vi "Vision Processing.vi"(4 "error in (no error)":errorcluster, 7 "Image Size":T5=enum."320x240") -> ()   [LabVIEW 2016]
doc: "This VI runs in parallel to other tasks. It gets images from the camera, processes them for color or shape and use that information to affect robot behavior."
uses:
  <vilib>/Rock Robotics/WPI/Camera/WPI_CameraImageSize.ctl
  Quick Vision/Typedefs/typedef_enum_ColorSpace.ctl
  <vilib>/Rock Robotics/WPI/Camera/WPI_CameraWhite Balance Values.ctl
  <vilib>/Rock Robotics/WPI/Camera/WPI_CameraExposure Values.ctl
  <vilib>/Rock Robotics/WPI/Camera/WPI_CameraFrameRate.ctl
  Robot Global Data.vi
panel:
  in  "Frame Rate (fps)":T1=15
  in  "Brightness":i32=50
  in  "Compression":i32=40
  in  "Exposure":T2=enum."Flicker-free 60 Hz"
  in  "White Balance":T3=enum."Fixed fluorescent 1"
  in  "ColorMask Low/High":u8[][](array[slide])=[[0, 124], [155, 255], [178, 245]] scale=0.0..255.0
  in  "Threshhold":i32=20
  in  "ColorSpace":T4
  out "Process FPS":dbl=7.231066612610667 format="%.1f"
  # "Modify Values\n\nthen\n\nEdit (menu):\n\nMake Current\nValues Default"
  # "Red\nHue\n\n\n\nGrn\nSat\n\n\n\nBlu\nLit"
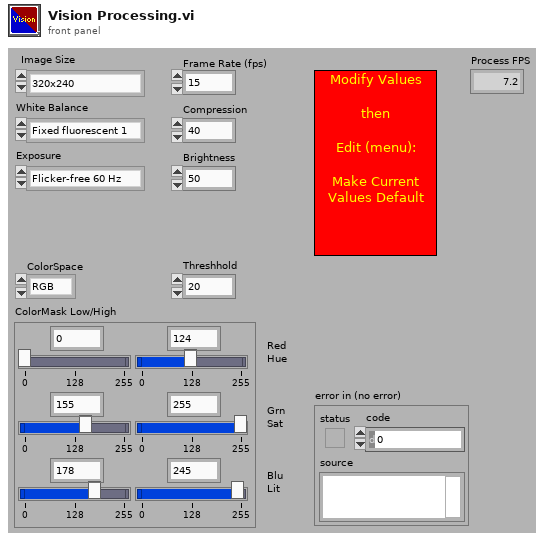
[diagram p1: front panel]
types:
  T1 = typedef "WPI_CameraFrameRate.ctl" = u32
  T2 = typedef "WPI_CameraExposure Values.ctl" = enum16{"Auto", "Flicker-free 50 Hz", "Flicker-free 60 Hz", "Hold current", "Custom"}
  T3 = typedef "WPI_CameraWhite Balance Values.ctl" = enum16{"Auto", "Fixed indoor", "Fixed outdoor 1", "Fixed outdoor 2", "Fixed fluorescent 1", "Fixed fluorescent 2", "Hold current", "Custom"}
  T4 = typedef "typedef_enum_ColorSpace.ctl" = enum16{"RGB", "HSL"}
  T5 = typedef "WPI_CameraImageSize.ctl" = enum16{"640x480", "320x240", "160x120", "Custom"}
  T6 = typedef "Image Type" = u32
  T7 = typedef "WPI_CameraDevRef.ctl" = cluster{"Camera Address":string, "CameraStatus":errorcluster}
  T8 = typedef "IMAQ Image.ctl" = refnum<image>
  T9 = typedef "typedef_cluster_Object Params.ctl" = cluster{"Dist_ft":dbl, "Deg_Rt":dbl, "Deg_Up":dbl, "Cam_FPS":dbl}
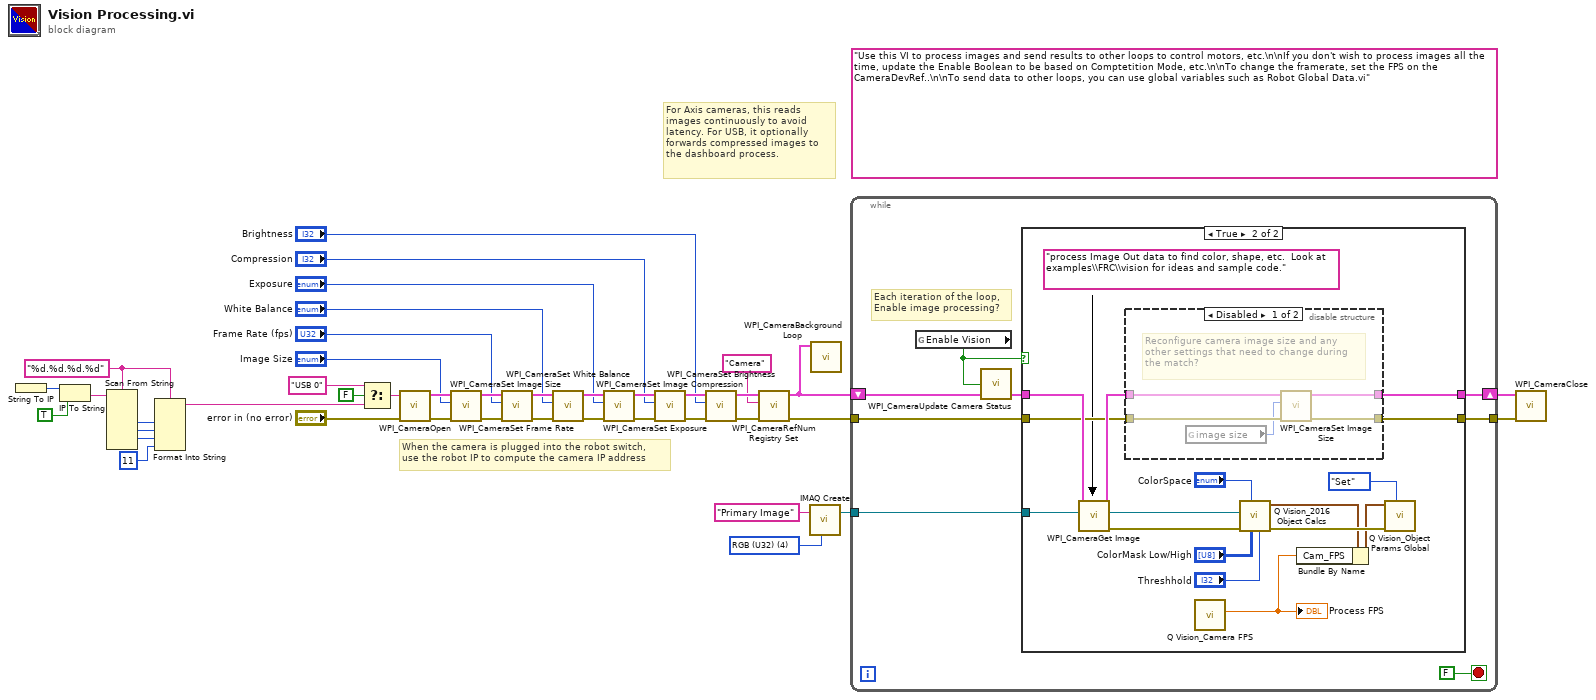
[diagram p0: block diagram]
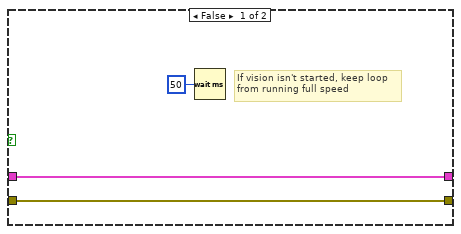
[diagram p2: hidden frame]
diagram:
  w14 = "%d.%d.%d.%d" ("format string")
  (unwired) "Use this VI to process images and send results to other loops to control motors, etc.\n\nIf you don't wish to process images all the time, update the Enable Boolean to be based on Comptetition Mode, etc.\n\nTo change the framerate, set the FPS on the CameraDevRef..\n\nTo send data to other loops, you can use global variables such as Robot Global Data.vi"
  w41 = T6 4 items=["Grayscale (U8)", "Grayscale (I16)", "Grayscale (SGL)", "Complex (CSG)", "RGB (U32)", "HSL (U32)", "RGB (U64)"] ("Image Type")
  # "When the camera is plugged into the robot switch,\nuse the robot IP to compute the camera IP address"
  # "For Axis cameras, this reads\nimages continuously to avoid\nlatency. For USB, it optionally\nforwards compressed images to\nthe dashboard process."
  n1 = String To IP() -> (0:w21:u32)  [unwired: 1 in]
  n2 = IP To String(1:TRUE ("dot notation? (F)"), 2:w21) -> (0:w19:string)
  n3 = Scan From String(format string=w14, input string=w19) -> (output 1=w18:i32, output 2=w17:i32, output 3=w16:i32)  [unwired: 7 in, 3 out]
  n4 = Format Into String(format string=w14, w18, w17, w16, 11 ("Compression")) -> (resulting string=w9:string)  [unwired: 2 in, 1 out]
  n5 = Select(t="USB 0" ("format string"), s=FALSE ("dot notation? (F)"), f=w9) -> (s? t:f=w7:string)
  n6 = call <vilib>:"WPI_CameraOpen.vi"("error in (no error)"="error in (no error)", "Camera Address"=w7) -> ("error out"=w32:errorcluster, "CameraDevRef"=w33:T7)  [unwired: 8 out]
  n7 = call <vilib>:"WPI_CameraSet Image Size.vi"("error in (no error)"=w32, "Image Size"="Image Size", "CameraDevRef"=w33) -> ("error out"=w31:errorcluster, "CameraDevRef Out"=w34:T7)  [unwired: 1 in, 6 out]
  n8 = call <vilib>:"WPI_CameraSet Frame Rate.vi"("error in (no error)"=w31, "Frame Rate (fps)"="Frame Rate (fps)", "CameraDevRef"=w34) -> ("error out"=w30:errorcluster, "CameraDevRef Out"=w36:T7)  [unwired: 7 out]
  n9 = call <vilib>:"WPI_CameraSet White Balance.vi"("error in (no error)"=w30, "White Balance"="White Balance", "CameraDevRef"=w36) -> ("error out"=w29:errorcluster, "CameraDevRef Out"=w35:T7)  [unwired: 1 in, 6 out]
  n10 = call <vilib>:"WPI_CameraSet Exposure.vi"("error in (no error)"=w29, "Exposure"="Exposure", "CameraDevRef"=w35) -> ("error out"=w28:errorcluster, "CameraDevRef Out"=w38:T7)  [unwired: 1 in, 6 out]
  n11 = call <vilib>:"WPI_CameraSet Image Compression.vi"("error in (no error)"=w28, "Compression"="Compression", "CameraDevRef"=w38) -> ("error out"=w27:errorcluster, "CameraDevRef Out"=w37:T7)  [unwired: 7 out]
  n12 = call <vilib>:"WPI_CameraSet Brightness.vi"("error in (no error)"=w27, "Brightness"="Brightness", "CameraDevRef"=w37) -> ("error out"=w25:errorcluster, "CameraDevRef Out"=w26:T7)  [unwired: 7 out]
  n13 = call <vilib>:"WPI_CameraRefNum Registry Set.vi"("error in (no error)"=w25, "refnum name"="Camera", "CameraDevRef"=w26) -> ("error out"=w6:errorcluster, "CameraDevRef"=w13:T7)  [unwired: 1 in, 6 out]
  n14 = call "IMAQ Create"("Image Name"="Primary Image", "Image Type"=w41) -> ("New Image"=w39:T8)  [unwired: 2 in, 2 out]
  n15 = call <vilib>:"WPI_CameraBackground Loop.vi"("CameraDevRef"=w13) -> ()  [unwired: 11 in]
  n16 = while {
    shift-right: [w49] -> w11
    shift-left: w13 -> [w47]
    tunnel: w39 -> [w48]
    tunnel: w6 -> [w44]
    tunnel: [w43] -> w5
    stop <- FALSE stop-if-true
    # "Each iteration of the loop,\nEnable image processing?"
    n17 = global read "Robot Global Data.vi" "Enable Vision"() -> (w45:bool)
    n18 = call <vilib>:"WPI_CameraUpdate Camera Status.vi"("CameraDevRef In"=w47, "Enable Vision"=w45) -> ("CameraDevRef Out"=w46:T7)  [unwired: 3 in]
    n19 = case shown="True" w45 {
      tunnel: w48 -> [_ w67]
      tunnel: [w52 w68] -> w49
      tunnel: w46 -> [w52 w66]
      tunnel: w44 -> [w50 w53]
      tunnel: [w50 w54] -> w43
      frame False {
        # "If vision isn't started, keep loop\nfrom running full speed"
        n20 = Wait (ms)(milliseconds to wait=u32 50) -> ()  [unwired: 1 out]
      }
      frame True {
        (unwired) "process Image Out data to find color, shape, etc.  Look at examples\\FRC\\vision for ideas and sample code."
        n21 = call <vilib>:"WPI_CameraGet Image.vi"("Image"=w67, "CameraDevRef"=w66) -> ("error out"=w62:errorcluster, "Image Out"=w63:T8, "CameraDevRef Out"=w65:T7)  [unwired: 1 in, 6 out]
        n22 = disable-structure shown="Disabled" {
          disable-tunnel: [w73 w75] -> w68
          disable-tunnel: w65 -> [w72 w75]
          disable-tunnel: [w70 w74] -> w54
          disable-tunnel: w53 -> [w71 w74]
          frame Disabled {
            # "Reconfigure camera image size and any\nother settings that need to change during\nthe match?"
            n23 = global read "Robot Global Data.vi" "image size"() -> (w69:T5)
            n24 = call <vilib>:"WPI_CameraSet Image Size.vi"("error in (no error)"=w71, "Image Size"=w69, "CameraDevRef"=w72) -> ("error out"=w70:errorcluster, "CameraDevRef Out"=w73:T7)  [unwired: 1 in, 6 out]
          }
          frame Enabled {
          }
        }
        n25 = call "Q Vision_Camera FPS.vi"() -> ("Avg_FPS"=w55:dbl)  [unwired: 10 in, 1 out]
        "Process FPS" <- w55
        n26 = call "Q Vision_2016 Object Calcs.vi"("Threshhold"="Threshhold", "ColorMask Low/High"="ColorMask Low/High", "ColorSpace"="ColorSpace", "error in (no error)"=w62, "Image in"=w63) -> ("error out"=w61:errorcluster, "Object Params out"=w57:T9)  [unwired: 5 in]
        n27 = Bundle By Name(cluster=w57, "Cam_FPS"=w55) -> (w56:T9)
        n28 = call "Q Vision_Object Params Global.vi"("Action"=enum16{"Get", "Set"}."Set", "error in (no error)"=w61, "Object Params in"=w56) -> ()  [unwired: 7 in, 2 out]
      }
    }
  }
  n29 = call <vilib>:"WPI_CameraClose.vi"("error in (no error)"=w5, "CameraDevRef"=w11) -> ()  [unwired: 10 out]
